vi "Get Created Attributes.vi"(10 "Alias":string, 11 "Actor in":refnum<class "Actor.lvclass">) -> (1 "Is Found":bool, 2 "Created Attributes":refnum<class "Attributes.lvclass">)   [LabVIEW 2020, in "jettl.lvlib" / "Actor.lvlib" / "Actor.lvclass"]
uses:
  Actor.lvclass
  Attributes/Attributes/Attributes.lvclass
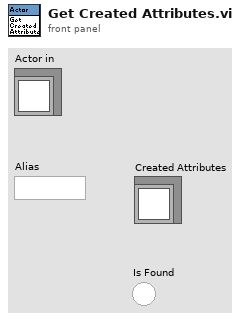
[diagram p1: front panel]
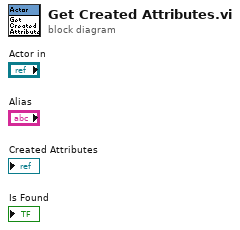
[diagram p0: block diagram]
diagram:
